vi "UART Open.vi"(8 "error in (no error)":errorcluster, 11 "VISA resource name in":refnum<visa-resource-name>) -> (0 "error out":errorcluster, 3 "VISA resource name out":refnum<visa-resource-name>)   [LabVIEW 2021, in "UART.lvlib"]
doc: "Opens the reference to one or more Universal Asynchronous Receiver/Transmitter (UART) channels. You must open a reference before you use a UART channel to access the VISA VIs and functions that communicate with devices connected to a serial port."
uses:
  <vilib>/myRIO/Instrument Drivers/Onboard IO/UART/UART.lvlib
  <vilib>/myRIO/Common/Instrument Driver Framework/ELVIS III v1.0/UART/vis/ELVIS III v1.0 Reserve UART.vi
  <vilib>/myRIO/Common/Instrument Driver Framework/ELVIS III v1.0/UART/vis/ELVIS III v1.0 Build MUX Configuration UART.vi
  <vilib>/Utility/error.llb/Error Cluster From Error Code.vi
  <vilib>/myRIO/Common/Instrument Driver Framework/ELVIS III v1.0/ELVIS III v1.1 Open.vi
  <vilib>/myRIO/Common/Instrument Driver Framework/ELVIS III v1.0/Resource Manager/vis/ELVIS III v1.0 Reserve Channel List.vi
  <vilib>/myRIO/Common/Instrument Driver Framework/ELVIS III v1.0/UART/vis/ELVIS III v1.0 Configure UART.vi
  <vilib>/myRIO/Common/Instrument Driver Framework/myRIO v1.0/myRIO v1.0 Close.vi
  <vilib>/userdefined/High Color/nirio_resource_hc.ctl
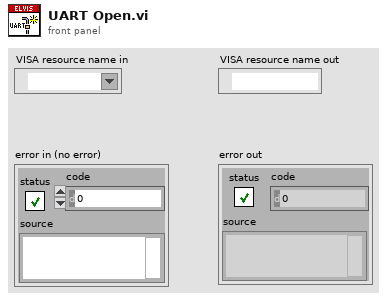
[diagram p1: front panel]
types:
  T1 = typedef "nirio_resource_hc.ctl" = tag
  T2 = typedef "Hardware Version Enum.ctl" = enum16{"Unknown", "myRIO-1900", "myRIO-1950", "roboRIO", "NI ELVIS RIO CM", "ELVIS III"}
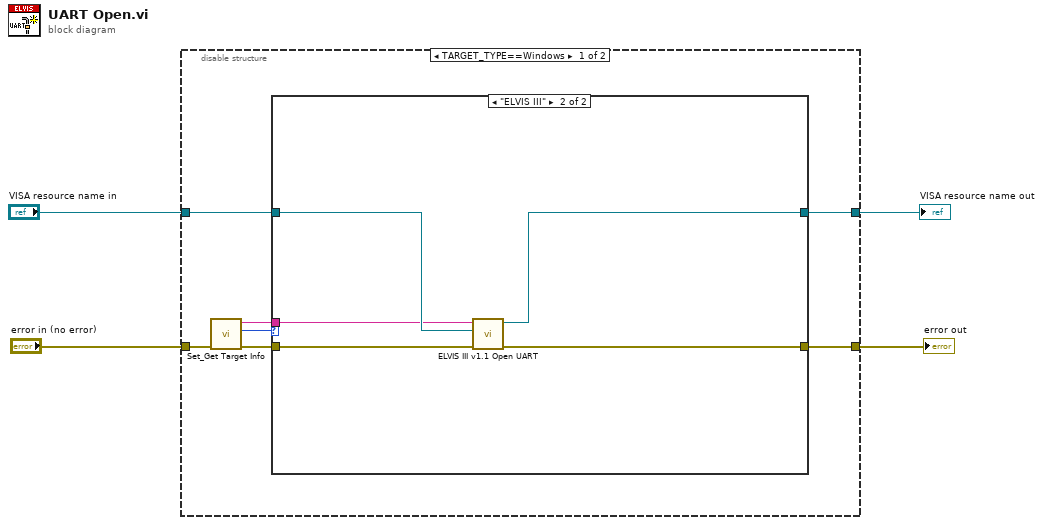
[diagram p0: block diagram]
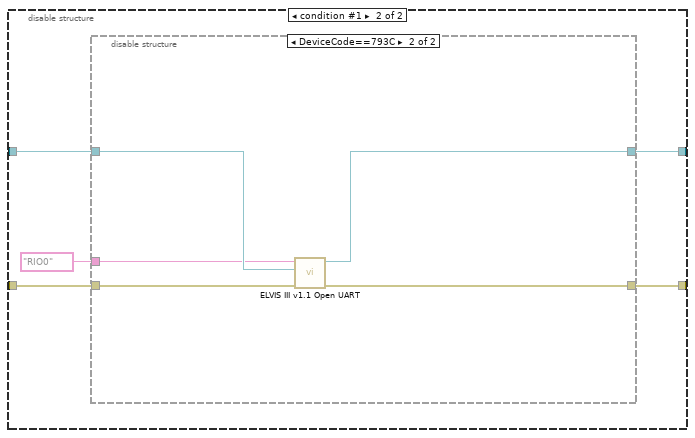
[diagram p3: hidden frame]
diagram:
  n1 = disable-structure shown="TARGET_TYPE==Windows" {
    disable-tunnel: "VISA resource name in" -> [w9 w22]
    disable-tunnel: [w8 w23] -> w3
    disable-tunnel: "error in (no error)" -> [w7 w20]
    disable-tunnel: [w5 w21] -> w1
    frame condition #0 (active) {
      n2 = call <vilib>:"Set_Get Target Info.vi"("error in (no error)"=w7) -> ("error out"=w6:errorcluster, "Hardware Version"=w10:T2, "IP Address"=w11:string)  [unwired: 8 in]
      n3 = case shown="\"ELVIS III\"" w10 {
        tunnel: w11 -> [_ w16]
        tunnel: w9 -> [w13 w17]
        tunnel: [w13 w18] -> w8
        tunnel: w6 -> [w12 w15]
        tunnel: [w12 w14] -> w5
        frame "Unknown", Default {
        }
        frame "ELVIS III" {
          n4 = call <vilib>:"ELVIS III v1.1 Open UART.vi"("error in (no error)"=w15, "VISA resource name in"=w17, "Resource name"=w16) -> ("error out"=w14:errorcluster, "VISA resource name"=w18:refnum<visa-resource-name>)  [unwired: 7 in]
        }
      }
    }
    frame condition #1 {
      n5 = disable-structure shown="DeviceCode==793C" {
        disable-tunnel: [w25 w30] -> w23
        disable-tunnel: w22 -> [w25 w28]
        disable-tunnel: [w24 w29] -> w21
        disable-tunnel: w20 -> [w24 w26]
        disable-tunnel: T1 "RIO0" ("Resource name") -> [_ w27]
        frame condition #0 (active) {
        }
        frame condition #1 {
          n6 = call <vilib>:"ELVIS III v1.1 Open UART.vi"("error in (no error)"=w26, "VISA resource name in"=w28, "Resource name"=w27) -> ("error out"=w29:errorcluster, "VISA resource name"=w30:refnum<visa-resource-name>)  [unwired: 7 in]
        }
      }
    }
  }
  "VISA resource name out" <- w3
  "error out" <- w1
